vi "Format Event Timing Windows into Table.vi"(11 "Windows":T1[](array[typedef])) -> (3 "Table":string[][](array[string]))   [LabVIEW 2015, in "Engine Simulation Toolkit System Explorer.lvlib"]
uses:
  Engine Simulation Toolkit System Explorer.lvlib
  Event Timing Window.ctl
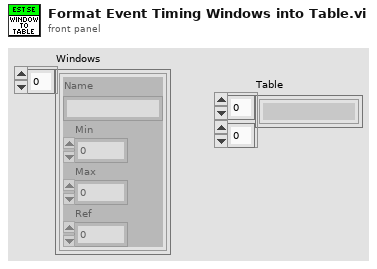
[diagram p1: front panel]
types:
  T1 = typedef "Engine Simulation Toolkit System Explorer.lvlib/Event Timing Window.ctl" = cluster{"Name":string, "Min":dbl, "Max":dbl, "Ref":dbl}
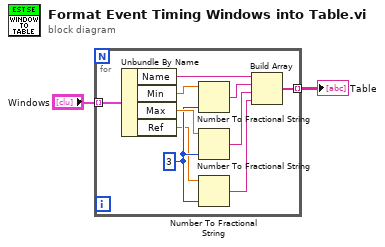
[diagram p0: block diagram]
diagram:
  n1 = for {
    tunnel: "Windows" -> [w12] mode=indexing
    tunnel: [w6] -> w1 mode=indexing
    w5 = i16 3 ("precision (6)")
    n2 = Unbundle By Name(w12) -> ("Name"=w9:string, "Min"=w11:dbl, "Max"=w10:dbl, "Ref"=w4:dbl)
    n3 = Number To Fractional String(number=w11, precision (6)=w5) -> (F-format string=w8:string)  [unwired: 2 in]
    n4 = Number To Fractional String(number=w10, precision (6)=w5) -> (F-format string=w7:string)  [unwired: 2 in]
    n5 = Number To Fractional String(number=w4, precision (6)=w5) -> (F-format string=w3:string)  [unwired: 2 in]
    n6 = Build Array(w9, w8, w7, w3) -> (w6:string[])
  }
  "Table" <- w1
